vi "AutoLin Eingang Aufsplitten.vi"(8 "error in (no error)":errorcluster caption="Fehler (Eingang, kein Fehler)", 11 "Eingabetabelle":T1) -> (0 "error out":errorcluster caption="Fehler (Ausgang)", 1 "Sollwerte":dbl[](array[numeric]), 2 "Rohwerte":dbl[](array[numeric]), 3 "Eingabetabelle out":T1, 4 "Linearisiert":dbl[](array[numeric]))   [LabVIEW 2020, in "Linearisierung v2.lvlib"]
uses:
  Linearisierung v2.lvlib
  Eingabetabelle.ctl
  Allgemein/allgemeine Sub-VIs.lvlib
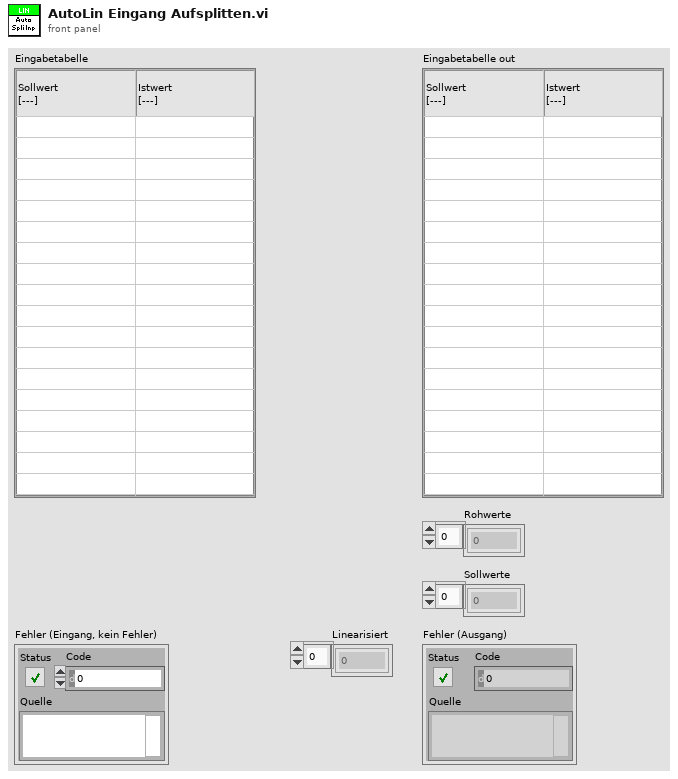
[diagram p1: front panel]
types:
  T1 = typedef "Linearisierung v2.lvlib/Eingabetabelle.ctl" = string[][]
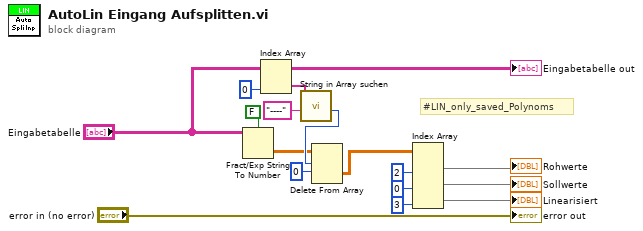
[diagram p0: block diagram]
diagram:
  # "#LIN_only_saved_Polynoms"
  n1 = Fract/Exp String To Number(use system decimal point (T)=FALSE ("Systemdezimalzeichen verwenden (T)"), string="Eingabetabelle") -> (number=w6:dbl[][])  [unwired: 2 in, 1 out]
  n2 = Index Array(array="Eingabetabelle", index (col)=0 ("Deaktivierter Index (Spalte)")) -> (element=w8:string[])  [unwired: 1 in]
  n3 = call "String in Array suchen.vi"("Nach String/Zeichen suchen (-)"="----", "String-Array"=w8) -> ("Index"=w9:i32)  [unwired: 7 in, 2 out]
  n4 = Delete From Array(array=w6, length=w9, index (row)=0 ("Index (Zeile)")) -> (deleted portion=w11:dbl[][])  [unwired: 1 in, 1 out]
  n5 = Index Array(array=w11, index (col) #1=2 ("Deaktivierter Index (Spalte)"), index (col) #2=0 ("Index (Spalte)"), index (col) #3=3 ("Index (Spalte)")) -> (element #1=→"Rohwerte":dbl[], element #2=→"Sollwerte":dbl[], element #3=→"Linearisiert":dbl[])  [unwired: 3 in]
  "Eingabetabelle out" <- "Eingabetabelle"
  "error out" <- "error in (no error)"
